vi "PIM Append Group Data Fields.vi"(10 "PIM Results":T1={"Measurement Cycles"=0, "Calibration State"=FALSE, "Data"=[], "PIM Test Parameters"={"Stimulus"={"C1 Pwr dBm"=43.0, "C2 Pwr dBm"=43.0, "Power Units"=enum."dBm", "Meas Type"=enum."Time", "C1 Freq MHz"=0.0, "C2 Freq MHz"=0.0, "Swept Freq Step"=0}, "Measure"={"IM Order"=0, "Direction"=0, "Averaging"=2, "ALC ON?"=TRUE, "Peak Hold?"=TRUE, "Peak last N"=0, "Ref Level dBm"=-100.0, "Ref Units"=enum."dBm", "Num Samples"=0, "Sample units"=enum."Sample(s)", "Update Rate (s)"=0.0, "DUT PORT"=enum."Port 1", "Percent (%)"=100}, "Display"={"Power Scale"={"yRange_min"=-160, "yRange_max"=-60}, "xRange_span"=1}}, "Peak IM Level"=0.0, "Instrument String"="", "Instrument Used"={"ixInstrument"=0, "sxInstrumentId"="", "sDriverId"="", "sDriverType"="", "sSerialNumber"="", "tLastCalibration"=timestamp(0 s since 1904-01-01), "tCalibrationDue"=timestamp(0 s since 1904-01-01), "sConfiguration"=""}} {"PIM Test Parameters"."Stimulus"."Swept Freq Step" items=[".2", ".4", "1.0", "2.0"]; "PIM Test Parameters"."Measure"."Averaging" items=["None", "Minimum", "Normal", "High", "Maximum"]; "PIM Test Parameters"."Measure"."Direction" items=["Reverse", "Forward", "Auxiliary"]; "PIM Test Parameters"."Measure"."IM Order" items=["3rd", "5th", "7th", "9th", "11th", "13th", "15th", "17th", "19th", "21st", "23rd", "25th", "27th", "29th", "31st", "33rd"]}, 11 "Fields In":T13[](array[typedef])) -> (3 "Fields Out":T13[](array[typedef]))   [LabVIEW 2011]
uses:
  server/database/Fields/Field Record.ctl
  server/database/Fields/Field DataTypes.ctl
  server/database/Fields/Field NextItem.ctl
  TypeDefs/PIM Test Results.ctl
  TypeDefs/PIM Test Parameters.ctl
  TypeDefs/PIM Stimulus Parameters.ctl
  SI.LIB/PIM.LIB/HW IO/PIM Sweep Step Size.ctl
  TypeDefs/PIM Measurement Parameters.ctl
  SI.LIB/PIM.LIB/HW IO/IMOrder.ctl
  SI.LIB/PIM.LIB/HW IO/MeasMode.ctl
  SI.LIB/PIM.LIB/HW IO/HW Averaging.ctl
  TypeDefs/PIM Meas Units.ctl
  SI.LIB/PIM.LIB/HW IO/DUTport.ctl
  TypeDefs/PIM Display Parameters.ctl
  server/database/Stations/Instruments/Instrument Record.ctl
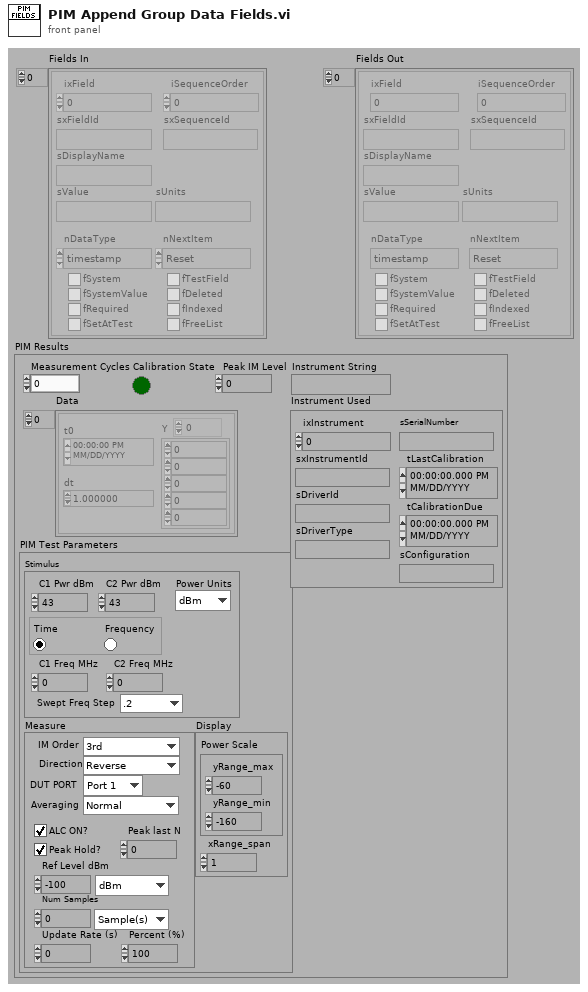
[diagram p1: front panel]
types:
  T1 = typedef "PIM Test Results.ctl" = cluster{"Measurement Cycles":i32, "Calibration State":bool, "Data":waveform(dbl)[], "PIM Test Parameters":T2, "Peak IM Level":dbl, "Instrument String":string, "Instrument Used":T12}
  T2 = typedef "PIM Test Parameters.ctl" = cluster{"Stimulus":T3, "Measure":T5, "Display":T11}
  T3 = typedef "PIM Stimulus Parameters.ctl" = cluster{"C1 Pwr dBm":dbl, "C2 Pwr dBm":dbl, "Power Units":enum16{"dBm", "Watts"}, "Meas Type":enum32{"Time", "Frequency"}, "C1 Freq MHz":dbl, "C2 Freq MHz":dbl, "Swept Freq Step":T4}
  T4 = typedef "PIM Sweep Step Size.ctl" = u16
  T5 = typedef "PIM Measurement Parameters.ctl" = cluster{"IM Order":T6, "Direction":T7, "Averaging":T8, "ALC ON?":bool, "Peak Hold?":bool, "Peak last N":u32, "Ref Level dBm":dbl, "Ref Units":enum16{"dBm", "dBc"}, "Num Samples":u32, "Sample units":T9, "Update Rate (s)":dbl, "DUT PORT":T10, "Percent (%)":u8}
  T6 = typedef "IMOrder.ctl" = u8
  T7 = typedef "MeasMode.ctl" = u16
  T8 = typedef "HW Averaging.ctl" = u16
  T9 = typedef "PIM Meas Units.ctl" = enum16{"Sample(s)", "Second(s)", "Sweep(s)"}
  T10 = typedef "DUTport.ctl" = enum16{"Port 1", "Port 2"}
  T11 = typedef "PIM Display Parameters.ctl" = cluster{"Power Scale":cluster{"yRange_min":i32, "yRange_max":i32}, "xRange_span":u32}
  T12 = typedef "Instrument Record.ctl" = cluster{"ixInstrument":i32, "sxInstrumentId":string, "sDriverId":string, "sDriverType":string, "sSerialNumber":string, "tLastCalibration":timestamp, "tCalibrationDue":timestamp, "sConfiguration":string}
  T13 = typedef "Field Record.ctl" = cluster{"ixField":i32, "iSequenceOrder":i32, "sxFieldId":string, "sxSequenceId":string, "sDisplayName":string, "sValue":string, "sUnits":string, "nDataType":T14, "nNextItem":T15, "fSystem":bool, "fSystemValue":bool, "fRequired":bool, "fSetAtTest":bool, "fTestField":bool, "fDeleted":bool, "fIndexed":bool, "fFreeList":bool}
  T14 = typedef "Field DataTypes.ctl" = enum32{"text", "numeric", "list", "timestamp", "boolean"}
  T15 = typedef "Field NextItem.ctl" = enum32{"Reset", "Retain", "Auto-Increment"}
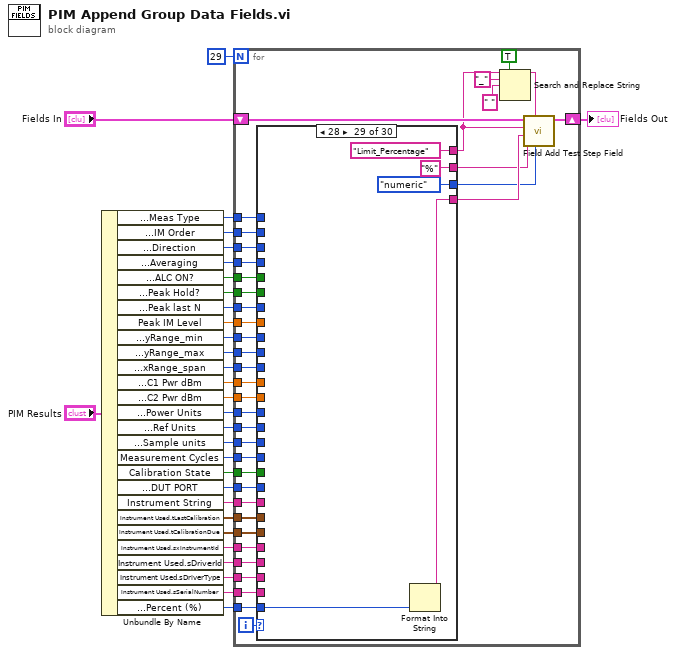
[diagram p0: block diagram]
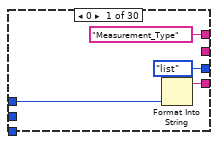
[diagram p2: hidden frame]
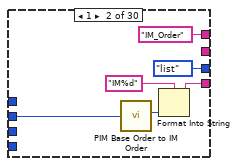
[diagram p3: hidden frame]
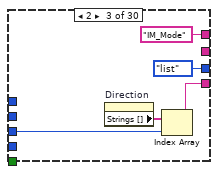
[diagram p4: hidden frame]
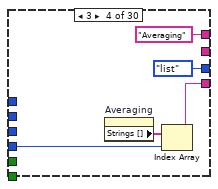
[diagram p5: hidden frame]
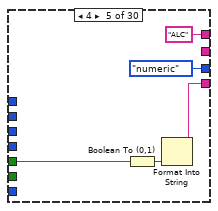
[diagram p6: hidden frame]
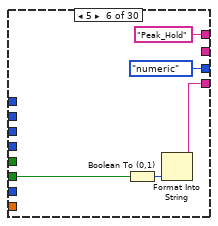
[diagram p7: hidden frame]
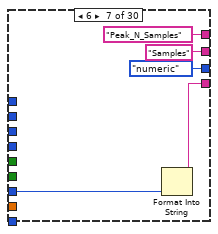
[diagram p8: hidden frame]
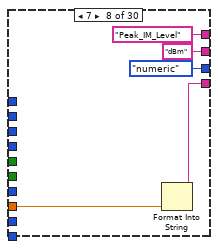
[diagram p9: hidden frame]
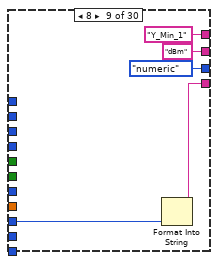
[diagram p10: hidden frame]
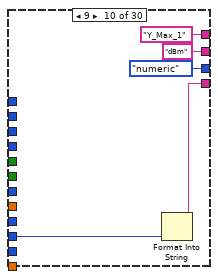
[diagram p11: hidden frame]
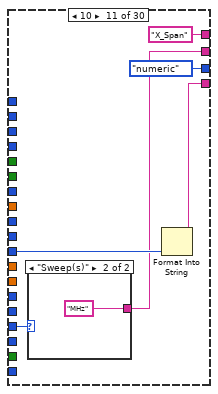
[diagram p12: hidden frame]
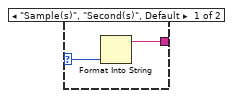
[diagram p13: hidden frame]
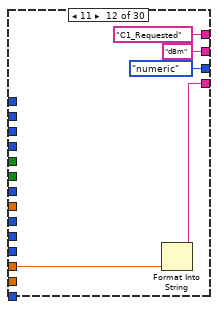
[diagram p14: hidden frame]
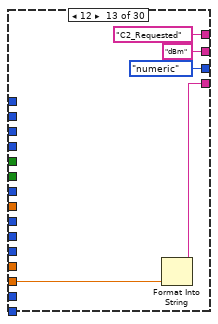
[diagram p15: hidden frame]
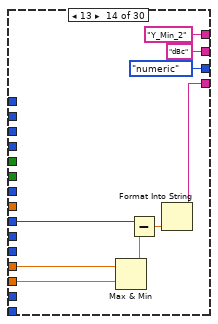
[diagram p16: hidden frame]
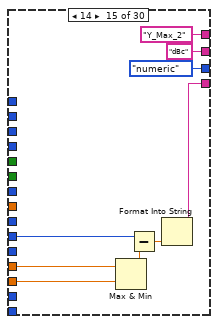
[diagram p17: hidden frame]
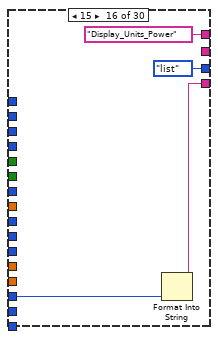
[diagram p18: hidden frame]
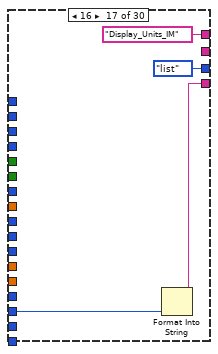
[diagram p19: hidden frame]
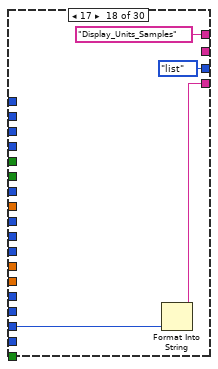
[diagram p20: hidden frame]
diagram:
  n1 = Unbundle By Name("PIM Results") -> ("PIM Test Parameters.Stimulus.Meas Type"=w27:enum32{"Time", "Frequency"}, "PIM Test Parameters.Measure.IM Order"=w26:T6, "PIM Test Parameters.Measure.Direction"=w25:T7, "PIM Test Parameters.Measure.Averaging"=w24:T8, "PIM Test Parameters.Measure.ALC ON?"=w23:bool, "PIM Test Parameters.Measure.Peak Hold?"=w22:bool, "PIM Test Parameters.Measure.Peak last N"=w21:u32, "Peak IM Level"=w20:dbl, "PIM Test Parameters.Display.Power Scale.yRange_min"=w12:i32, "PIM Test Parameters.Display.Power Scale.yRange_max"=w19:i32, "PIM Test Parameters.Display.xRange_span"=w18:u32, "PIM Test Parameters.Stimulus.C1 Pwr dBm"=w17:dbl, "PIM Test Parameters.Stimulus.C2 Pwr dBm"=w16:dbl, "PIM Test Parameters.Stimulus.Power Units"=w15:enum16{"dBm", "Watts"}, "PIM Test Parameters.Measure.Ref Units"=w14:enum16{"dBm", "dBc"}, "PIM Test Parameters.Measure.Sample units"=w13:T9, "Measurement Cycles"=w11:i32, "Calibration State"=w10:bool, "PIM Test Parameters.Measure.DUT PORT"=w9:T10, "Instrument String"=w2:string, "Instrument Used.tLastCalibration"=w8:timestamp, "Instrument Used.tCalibrationDue"=w7:timestamp, "Instrument Used.sxInstrumentId"=w6:string, "Instrument Used.sDriverId"=w5:string, "Instrument Used.sDriverType"=w4:string, "Instrument Used.sSerialNumber"=w3:string, "PIM Test Parameters.Measure.Percent (%)"=w1:u8)
  n2 = for {
    N: 29 -> [_]
    tunnel: w18 -> [w68]
    tunnel: w19 -> [w67]
    tunnel: w20 -> [w66]
    tunnel: w21 -> [w65]
    tunnel: w22 -> [w64]
    tunnel: w23 -> [w63]
    tunnel: w24 -> [w62]
    tunnel: w25 -> [w61]
    tunnel: w26 -> [w60]
    tunnel: w27 -> [w59]
    shift-right: [w52] -> w30
    shift-left: "Fields In" -> [w53]
    tunnel: w17 -> [w58]
    tunnel: w16 -> [w57]
    tunnel: w15 -> [w56]
    tunnel: w14 -> [w55]
    tunnel: w13 -> [w54]
    tunnel: w12 -> [w48]
    tunnel: w11 -> [w47]
    tunnel: w10 -> [w46]
    tunnel: w9 -> [w45]
    tunnel: w8 -> [w44]
    tunnel: w7 -> [w43]
    tunnel: w6 -> [w42]
    tunnel: w5 -> [w41]
    tunnel: w4 -> [w40]
    tunnel: w3 -> [w39]
    tunnel: w2 -> [w38]
    tunnel: w1 -> [w32]
    i -> [w69]
    n3 = case shown="28" w69 {
      tunnel: w68 -> [_ _ _ _ _ _ _ _ _ _ w123 _ _ _ _ _ _ _ _ _ _ _ _ _ _ _ _ _ _ _]
      tunnel: w67 -> [_ _ _ _ _ _ _ _ _ w118 _ _ _ _ w150 _ _ _ _ _ _ _ _ _ _ _ _ _ _ _]
      tunnel: w66 -> [_ _ _ _ _ _ _ w106 _ _ _ _ _ _ _ _ _ _ _ _ _ _ _ _ _ _ _ _ _ _]
      tunnel: w65 -> [_ _ _ _ _ _ w102 _ _ _ _ _ _ _ _ _ _ _ _ _ _ _ _ _ _ _ _ _ _ _]
      tunnel: w64 -> [_ _ _ _ _ w96 _ _ _ _ _ _ _ _ _ _ _ _ _ _ _ _ _ _ _ _ _ _ _ _]
      tunnel: w63 -> [_ _ _ _ w91 _ _ _ _ _ _ _ _ _ _ _ _ _ _ _ _ _ _ _ _ _ _ _ _ _]
      tunnel: w62 -> [_ _ _ w86 _ _ _ _ _ _ _ _ _ _ _ _ _ _ _ _ _ _ _ _ _ _ _ _ _ _]
      tunnel: w61 -> [_ _ w80 _ _ _ _ _ _ _ _ _ _ _ _ _ _ _ _ _ _ _ _ _ _ _ _ _ _ _]
      tunnel: w60 -> [_ w77 _ _ _ _ _ _ _ _ _ _ _ _ _ _ _ _ _ _ _ _ _ _ _ _ _ _ _ _]
      tunnel: w59 -> [w71 _ _ _ _ _ _ _ _ _ _ _ _ _ _ _ _ _ _ _ _ _ _ _ _ _ _ _ _ _]
      tunnel: ["Measurement_Type" ("Field_ID") "IM_Order" ("Field_ID") "IM_Mode" ("Field_ID") "Averaging" ("Field_ID") "ALC" ("Field_ID") "Peak_Hold" ("Field_ID") "Peak_N_Samples" ("Field_ID") "Peak_IM_Level" ("Field_ID") "Y_Min_1" ("Field_ID") "Y_Max_1" ("Field_ID") "X_Span" ("Field_ID") "C1_Requested" ("Field_ID") "C2_Requested" ("Field_ID") "Y_Min_2" ("Field_ID") "Y_Max_2" ("Field_ID") "Display_Units_Power" ("Field_ID") "Display_Units_IM" ("Field_ID") "Display_Units_Samples" ("Field_ID") "Cycles" ("Field_ID") "Calibration_Status" ("Field_ID") "DUT_Port" ("Field_ID") "Instrument_Devices_Used" ("Field_ID") "Instrument_Calibration_Date" ("Field_ID") "Instrument_Calibration_Due_Date" ("Field_ID") "Instrument_Name" ("Field_ID") "Instrument_Driver" ("Field_ID") "Instrument_Type" ("Field_ID") "Instrument_Serial_Number" ("Field_ID") "Limit_Percentage" ("Field_ID") _] -> w34
      tunnel: [Field_DataTypes."list" ("Data Type") Field_DataTypes."list" ("Data Type") Field_DataTypes."list" ("Data Type") Field_DataTypes."list" ("Data Type") Field_DataTypes."numeric" ("Data Type") Field_DataTypes."numeric" ("Data Type") Field_DataTypes."numeric" ("Data Type") Field_DataTypes."numeric" ("Data Type") Field_DataTypes."numeric" ("Data Type") Field_DataTypes."numeric" ("Data Type") Field_DataTypes."numeric" ("Data Type") Field_DataTypes."numeric" ("Data Type") Field_DataTypes."numeric" ("Data Type") Field_DataTypes."numeric" ("Data Type") Field_DataTypes."numeric" ("Data Type") Field_DataTypes."list" ("Data Type") Field_DataTypes."list" ("Data Type") Field_DataTypes."list" ("Data Type") Field_DataTypes."numeric" ("Data Type") Field_DataTypes."numeric" ("Data Type") Field_DataTypes."list" ("Data Type") Field_DataTypes."text" ("Data Type") Field_DataTypes."timestamp" ("Data Type") Field_DataTypes."timestamp" ("Data Type") Field_DataTypes."text" ("Data Type") Field_DataTypes."text" ("Data Type") Field_DataTypes."text" ("Data Type") Field_DataTypes."text" ("Data Type") Field_DataTypes."numeric" ("Data Type") Field_DataTypes."text" ("Data Type")] -> w50
      tunnel: [w70 w74 w81 w85 w93 w98 w103 w108 w113 w116 w124 w132 w137 w146 w155 w159 w163 w167 w171 w176 w180 w182 w185 w191 w195 w198 w201 w204 w210 _] -> w51
      tunnel: w58 -> [_ _ _ _ _ _ _ _ _ _ _ w131 _ w145 w154 _ _ _ _ _ _ _ _ _ _ _ _ _ _ _]
      tunnel: w57 -> [_ _ _ _ _ _ _ _ _ _ _ _ w136 w144 w153 _ _ _ _ _ _ _ _ _ _ _ _ _ _ _]
      tunnel: w56 -> [_ _ _ _ _ _ _ _ _ _ _ _ _ _ _ w158 _ _ _ _ _ _ _ _ _ _ _ _ _ _]
      tunnel: w55 -> [_ _ _ _ _ _ _ _ _ _ _ _ _ _ _ _ w162 _ _ _ _ _ _ _ _ _ _ _ _ _]
      tunnel: w54 -> [_ _ _ _ _ _ _ _ _ _ w121 _ _ _ _ _ _ w166 _ _ _ _ _ _ _ _ _ _ _ _]
      tunnel: [_ _ _ _ _ _ "Samples" ("Field_ID") "dBm" ("Field_ID") "dBm" ("Field_ID") "dBm" ("Field_ID") w120 "dBm" ("Field_ID") "dBm" ("Field_ID") "dBc" ("Field_ID") "dBc" ("Field_ID") _ _ _ _ _ _ _ _ _ _ _ _ _ "%" ("Field_ID") ""] -> w49
      tunnel: w48 -> [_ _ _ _ _ _ _ _ w111 _ _ _ _ w141 _ _ _ _ _ _ _ _ _ _ _ _ _ _ _ _]
      tunnel: w47 -> [_ _ _ _ _ _ _ _ _ _ _ _ _ _ _ _ _ _ w169 _ _ _ _ _ _ _ _ _ _ _]
      tunnel: w46 -> [_ _ _ _ _ _ _ _ _ _ _ _ _ _ _ _ _ _ _ w174 _ _ _ _ _ _ _ _ _ _]
      tunnel: w45 -> [_ _ _ _ _ _ _ _ _ _ _ _ _ _ _ _ _ _ _ _ w178 _ _ _ _ _ _ _ _ _]
      tunnel: w44 -> [_ _ _ _ _ _ _ _ _ _ _ _ _ _ _ _ _ _ _ _ _ _ w186 _ _ _ _ _ _ _]
      tunnel: w43 -> [_ _ _ _ _ _ _ _ _ _ _ _ _ _ _ _ _ _ _ _ _ _ _ w190 _ _ _ _ _ _]
      tunnel: w42 -> [_ _ _ _ _ _ _ _ _ _ _ _ _ _ _ _ _ _ _ _ _ _ _ _ w195 _ _ _ _ _]
      tunnel: w41 -> [_ _ _ _ _ _ _ _ _ _ _ _ _ _ _ _ _ _ _ _ _ _ _ _ _ w198 _ _ _ _]
      tunnel: w40 -> [_ _ _ _ _ _ _ _ _ _ _ _ _ _ _ _ _ _ _ _ _ _ _ _ _ _ w201 _ _ _]
      tunnel: w39 -> [_ _ _ _ _ _ _ _ _ _ _ _ _ _ _ _ _ _ _ _ _ _ _ _ _ _ _ w204 _ _]
      tunnel: w38 -> [_ _ _ _ _ _ _ _ _ _ _ _ _ _ _ _ _ _ _ _ _ w182 _ _ _ _ _ _ _ _]
      tunnel: w32 -> [_ _ _ _ _ _ _ _ _ _ _ _ _ _ _ _ _ _ _ _ _ _ _ _ _ _ _ _ w207 _]
      frame 0 {
        n4 = Format Into String(w71) -> (resulting string=w70:string)  [unwired: 3 in, 1 out]
      }
      frame 1 {
        n5 = call "PIM Base Order to IM Order.vi"("Base Order (0)"=w77) -> ("IM Order"=w75:u8)  [unwired: 5 out]
        n6 = Format Into String(format string="IM%d", w75) -> (resulting string=w74:string)  [unwired: 2 in, 1 out]
      }
      frame 2 {
        n7 = property on="Direction" class="Ring (strict)"() -> ("Strings []"=w82:string[])  [unwired: 2 in, 2 out]
        n8 = Index Array(array=w82, index=w80) -> (element=w81:string)
      }
      frame 3 {
        n9 = property on="Averaging" class="Ring (strict)"() -> ("Strings []"=w87:string[])  [unwired: 2 in, 2 out]
        n10 = Index Array(array=w87, index=w86) -> (element=w85:string)
      }
      frame 4 {
        n11 = Boolean To (0,1)(Boolean=w91) -> (0, 1=w90:i16)
        n12 = Format Into String(w90) -> (resulting string=w93:string)  [unwired: 3 in, 1 out]
      }
      frame 5 {
        n13 = Boolean To (0,1)(Boolean=w96) -> (0, 1=w95:i16)
        n14 = Format Into String(w95) -> (resulting string=w98:string)  [unwired: 3 in, 1 out]
      }
      frame 6 {
        n15 = Format Into String(w102) -> (resulting string=w103:string)  [unwired: 3 in, 1 out]
      }
      frame 7 {
        n16 = Format Into String(w106) -> (resulting string=w108:string)  [unwired: 3 in, 1 out]
      }
      frame 8 {
        n17 = Format Into String(w111) -> (resulting string=w113:string)  [unwired: 3 in, 1 out]
      }
      frame 9 {
        n18 = Format Into String(w118) -> (resulting string=w116:string)  [unwired: 3 in, 1 out]
      }
      frame 10 {
        n19 = case shown="\"Sweep(s)\"" w121 {
          selector: w121 -> [w127 _]
          tunnel: [w126 "MHz" ("Field_ID")] -> w120
          frame "Sample(s)", "Second(s)", Default {
            n20 = Format Into String(w127) -> (resulting string=w126:string)  [unwired: 3 in, 1 out]
          }
          frame "Sweep(s)" {
          }
        }
        n21 = Format Into String(w123) -> (resulting string=w124:string)  [unwired: 3 in, 1 out]
      }
      frame 11 {
        n22 = Format Into String(w131) -> (resulting string=w132:string)  [unwired: 3 in, 1 out]
      }
      frame 12 {
        n23 = Format Into String(w136) -> (resulting string=w137:string)  [unwired: 3 in, 1 out]
      }
      frame 13 {
        n24 = Max & Min(x=w145, y=w144) -> (max(x,y)=w143:dbl)  [unwired: 1 out]
        n25 = Subtract(x=w141, y=w143) -> (x-y=w142:dbl)
        n26 = Format Into String(w142) -> (resulting string=w146:string)  [unwired: 3 in, 1 out]
      }
      frame 14 {
        n27 = Max & Min(x=w154, y=w153) -> (max(x,y)=w152:dbl)  [unwired: 1 out]
        n28 = Subtract(x=w150, y=w152) -> (x-y=w151:dbl)
        n29 = Format Into String(w151) -> (resulting string=w155:string)  [unwired: 3 in, 1 out]
      }
      frame 15 {
        n30 = Format Into String(w158) -> (resulting string=w159:string)  [unwired: 3 in, 1 out]
      }
      frame 16 {
        n31 = Format Into String(w162) -> (resulting string=w163:string)  [unwired: 3 in, 1 out]
      }
      frame 17 {
        n32 = Format Into String(w166) -> (resulting string=w167:string)  [unwired: 3 in, 1 out]
      }
      frame 18 {
        n33 = Format Into String(w169) -> (resulting string=w171:string)  [unwired: 3 in, 1 out]
      }
      frame 19 {
        n34 = Boolean To (0,1)(Boolean=w174) -> (0, 1=w173:i16)
        n35 = Format Into String(w173) -> (resulting string=w176:string)  [unwired: 3 in, 1 out]
      }
      frame 20 {
        n36 = Format Into String(w178) -> (resulting string=w180:string)  [unwired: 3 in, 1 out]
      }
      frame 21 {
      }
      frame 22 {
        n37 = To Double Precision Float(number=w186) -> (double precision float=w187:dbl)
        n38 = Format Into String(w187) -> (resulting string=w185:string)  [unwired: 3 in, 1 out]
      }
      frame 23 {
        n39 = To Double Precision Float(number=w190) -> (double precision float=w192:dbl)
        n40 = Format Into String(w192) -> (resulting string=w191:string)  [unwired: 3 in, 1 out]
      }
      frame 24 {
      }
      frame 25 {
      }
      frame 26 {
      }
      frame 27 {
      }
      frame 28 {
        n41 = Format Into String(w207) -> (resulting string=w210:string)  [unwired: 3 in, 1 out]
      }
      frame Default {
      }
    }
    n42 = Search and Replace String(replace all?=TRUE ("replace all? (F)"), input string=w34, search string="_", replace string=" " ("replace string (\"\")")) -> (result string=w33:string)  [unwired: 1 in, 6 out]
    n43 = call "Field Add Test Step Field.vi"("nDataType"=w50, "sDisplayName"=w33, "sUnits"=w49, "sValue"=w51, "sxFieldId"=w34, "Fields In"=w53) -> ("Fields Out"=w52:T13[])  [unwired: 5 out]
  }
  "Fields Out" <- w30
